vi "Check Cache.vi"(10 "Hash":string, 11 "Probe Cache Folder":path) -> (2 "Create New Probe VI?":bool)   [LabVIEW 2019, in "GOOP Probe.lvlib"]
uses:
  GOOP Probe.lvlib
  <vilib>/Utility/config.llb/NI_LVConfig.lvlib
  <vilib>/Utility/config.llb/Read Key (String).vi
  <vilib>/Utility/config.llb/Write Key (String).vi
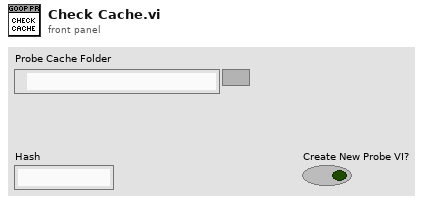
[diagram p1: front panel]
types:
  T1 = typedef "NI_LVConfig.lvlib/Config Data RefNum.ctl" = refnum<k1>
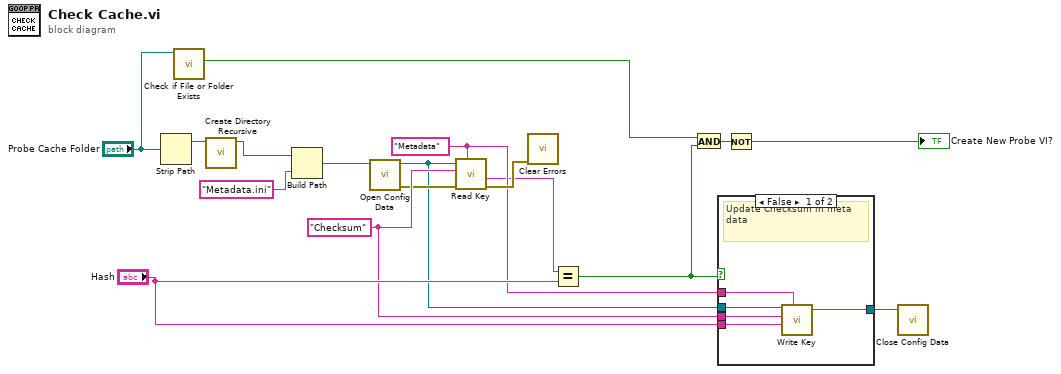
[diagram p0: block diagram]
diagram:
  w14 = "Metadata" ("section")
  w9 = "Checksum" ("key")
  n1 = Strip Path(path="Probe Cache Folder") -> (stripped path=w2:path)  [unwired: 1 out]
  n2 = call <vilib>:"Check if File or Folder Exists.vi"("path"="Probe Cache Folder") -> ("file or folder exists?"=w4:bool)  [unwired: 8 in, 2 out]
  n3 = call <vilib>:"Create Directory Recursive.vi"("directory"=w2) -> ("directory copy"=w16:path)  [unwired: 4 in, 2 out]
  n4 = Build Path(base path=w16, name or relative path="Metadata.ini" ("key")) -> (appended path=w11:path)
  n5 = call <vilib>:"Open Config Data.vi"("configuration file path"=w11) -> ("error out"=w8:errorcluster, "refnum"=w7:T1)  [unwired: 8 in, 1 out]
  n6 = call-poly <vilib>:"Read Key.vi"("section"=w14, "error in (no error)"=w8, "key"=w9, "refnum"=w7) -> ("error out"=w15:errorcluster, "value"=w12:string)  [unwired: 4 in, 2 out]
  n7 = call <vilib>:"Clear Errors.vi"("error in (no error)"=w15) -> ()  [unwired: 5 in, 2 out]
  n8 = Equal?(x=w12, y="Hash") -> (x = y?=w6:bool)
  n9 = And(x=w4, y=w6) -> (x .and. y?=w5:bool)
  n10 = case shown="False" w6 {
    tunnel: w7 -> [w22 w23]
    tunnel: w9 -> [w21 _]
    tunnel: "Hash" -> [w20 _]
    tunnel: [w19 w23] -> w13
    tunnel: w14 -> [w18 _]
    frame False {
      # "Update Checksum in meta data"
      n11 = call-poly <vilib>:"Write Key.vi"("section"=w18, "value"=w20, "key"=w21, "refnum"=w22) -> ("refnum out"=w19:T1)  [unwired: 5 in, 2 out]
    }
    frame True {
    }
  }
  n12 = Not(x=w5) -> (.not. x?=→"Create New Probe VI?":bool)
  n13 = call <vilib>:"Close Config Data.vi"("refnum"=w13) -> ()  [unwired: 9 in, 2 out]
